vi "Unflatten Value.vi"(8 "error in (no error)":errorcluster, 10 "Value":string, 11 "Boolean in":refnum<class "Persistence.lvclass">) -> (0 "error out":errorcluster, 3 "Boolean out":refnum<class "Persistence.lvclass">)   [LabVIEW 2017, in "Custom Type Test Executive.lvlib" / "Persistence.lvclass"]
uses:
  <vilib>/gpm_packages/@cs/test-executive/Source/Custom Type Test Executive/Persistence Data Type/Persistence.lvclass
  <vilib>/gpm_packages/@cs/persistence/source/IPersist/IPersist.lvclass
  <vilib>/gpm_packages/@cs/test-executive/Source/Custom Type Test Executive/Persistence Data Type/Persistence.lvclass/Persistence.ctl
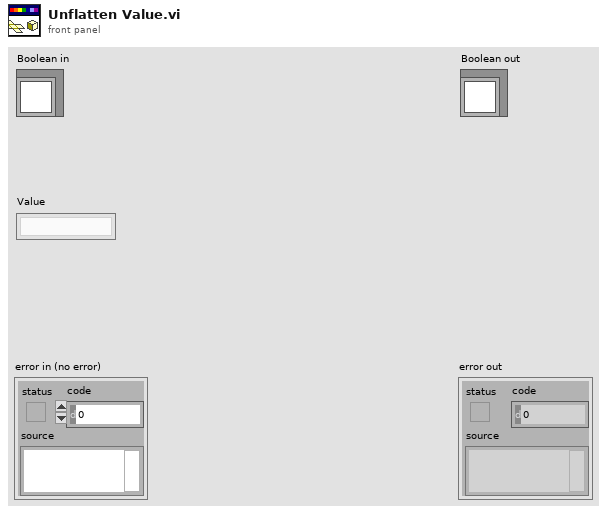
[diagram p1: front panel]
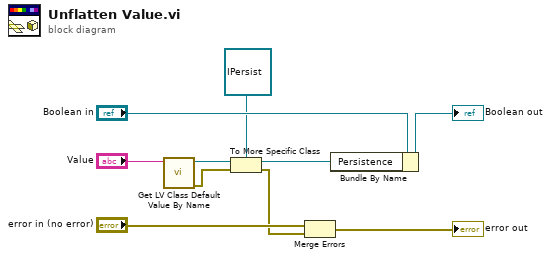
[diagram p0: block diagram]
diagram:
  n1 = call <vilib>:"Get LV Class Default Value By Name.vi"("class name"="Value") -> ("error out"=w1:errorcluster, "object"=w6:refnum<class>)  [unwired: 9 in]
  n2 = To More Specific Class(target class=refnum<class "IPersist.lvclass"> refnum ("Persistence"), reference=w6, error in=w1) -> (specific class reference=w4:refnum<class "IPersist.lvclass">, error out=w2:errorcluster)
  n3 = Merge Errors("error in (no error)", w2) -> (→"error out":errorcluster)
  n4 = Bundle By Name(cluster="Boolean in", "Persistence"=w4) -> (→"Boolean out":refnum<class "Persistence.lvclass">)
